vi "SupplyCHConfig.vi"(6 "CalArray":u8[](array[numeric]), 8 "error in (no error)":errorcluster caption="错误输入（无错误）", 9 "Voltage(V)":dbl=5.0, 10 "CH":enum16{"Positive", "Negative"}(ring), 11 "handle":u64) -> (0 "error out":errorcluster caption="错误输出", 2 "function return":i32, 3 "handle out":u64, 4 "CalArray out":u8[](array[numeric]))   [LabVIEW 2018]
doc: "Set pos. or neg. Supply voltage"
uses:
  InstrumentsPlayground.lvlib
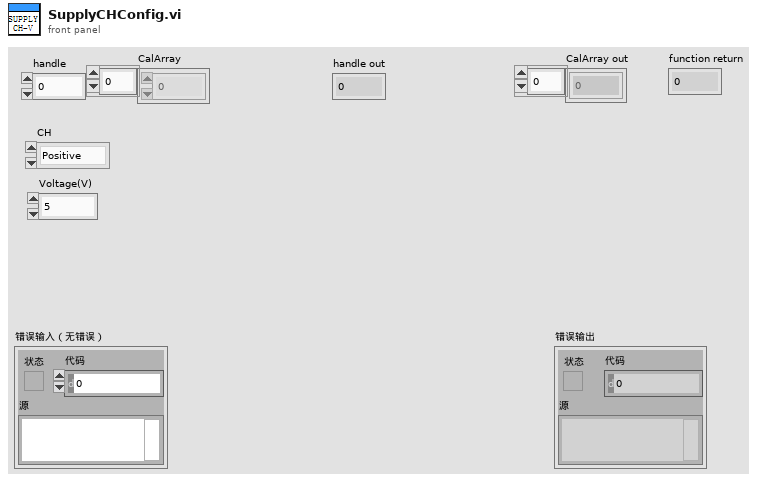
[diagram p1: front panel]
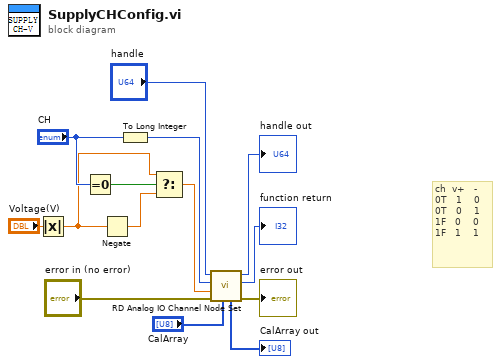
[diagram p0: block diagram]
diagram:
  # "ch  v+   -\n0T   1    0\n0T   0    1\n1F   0    0\n1F   1    1"
  n1 = Absolute Value(x="Voltage(V)") -> (abs(x)=w2:dbl)
  n2 = Equal To 0?(x="CH") -> (x = 0?=w1:bool)
  n3 = Negate(x=w2) -> (-x=w6:dbl)
  n4 = To Long Integer(number="CH") -> (32bit integer=w5:i32)
  n5 = Select(t=w2, s=w1, f=w6) -> (s? t:f=w8:dbl)
  n6 = call "RD Analog IO Channel Node Set.vi"("CalArray"="CalArray", "error in (no error)"="error in (no error)", "value"=w8, "ch"=w5, "handle"="handle") -> ("error out"=→"error out":errorcluster, "function return"=→"function return":i32, "handle out"=→"handle out":u64, "CalArray out"=→"CalArray out":u8[])  [unwired: 3 in]
